vi "Destruct.vi"(8 "Error in (no error)":errorcluster, 11 "LogWriterEmail in":refnum<class "LogWriterEmail.lvclass">) -> (0 "Error out":errorcluster, 2 "Array log out":T1[](array[typedef]) {"Priority" items=["EMERGENCY", "ALERT", "CRITICAL", "ERROR", "WARNING", "NOTICE", "INFO", "DEBUG"]})   [LabVIEW 2011, in "LogWriterEmail.lvclass"]
uses:
  LogWriterEmail.lvclass
  Log/LogCluster.ctl
  Log/PrioritiesRing.ctl
  LogWriterEmail.lvclass/LogWriterEmail.ctl
  LogWriterMock/LogWriterMock.lvclass
  Log/Log.lvclass
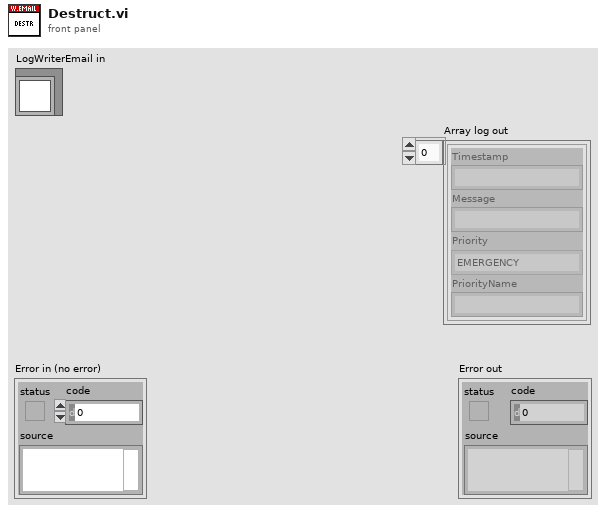
[diagram p1: front panel]
types:
  T1 = typedef "Log.lvclass/LogCluster.ctl" = cluster{"Timestamp":string, "Message":string, "Priority":T2, "PriorityName":string}
  T2 = typedef "Log.lvclass/PrioritiesRing.ctl" = u32
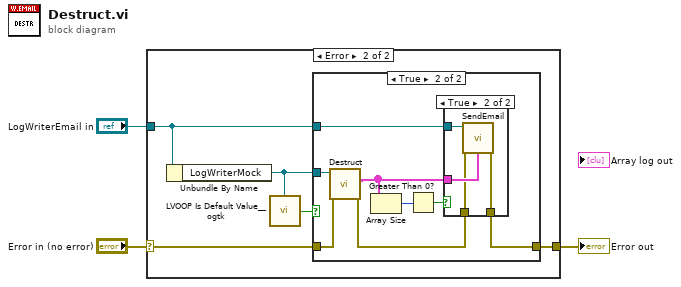
[diagram p0: block diagram]
diagram:
  n1 = case shown="Error" "Error in (no error)" {
    selector: "Error in (no error)" -> [w4 w8]
    tunnel: [w4 w7] -> w2
    tunnel: "LogWriterEmail in" -> [_ w9]
    frame No Error {
    }
    frame Error {
      n2 = Unbundle By Name(w9) -> ("LogWriterMock"=w6:refnum<class "LogWriterMock.lvclass">)
      n3 = call <userlib>:"LVOOP Is Default Value__ogtk.vi"("Object"=w6) -> ("Is Default Value?"=w5:bool)
      n4 = case shown="True" w5 {
        tunnel: w9 -> [_ w16]
        tunnel: w8 -> [w10 w14]
        tunnel: [w10 w11] -> w7
        tunnel: w6 -> [_ w13]
        frame False {
        }
        frame True {
          n5 = call-dynamic "Destruct.vi"("Error in (no error)"=w14, "LogWriterMock in"=w13) -> ("Error out"=w12:errorcluster, "Array log out"=w15:T1[])  [unwired: 8 in]
          n6 = Array Size(array=w15) -> (size(s)=w18:i32)
          n7 = Greater Than 0?(x=w18) -> (x > 0?=w17:bool)
          n8 = case shown="True" w17 {
            tunnel: w15 -> [_ w22]
            tunnel: w16 -> [_ w23]
            tunnel: w12 -> [w19 w21]
            tunnel: [w19 w20] -> w11
            frame False {
            }
            frame True {
              n9 = call "SendEmail.vi"("Error in (no error)"=w21, "Array log in"=w22, "LogWriterEmail in"=w23) -> ("Error out"=w20:errorcluster)  [unwired: 7 in, 1 out]
            }
          }
        }
      }
    }
  }
  "Error out" <- w2
